vi "Search for Home (SubVI).vi"(9 "Home Mode":T1, 10 "Axis":i32, 11 ".NET Refnum in":refnum<k24>) -> (0 "error out":errorcluster)   [LabVIEW 2019, in "ESP301.lvlib"]
uses:
  ESP301.lvlib
  Newport.ESP301.CommandInterface
  Home Mode.ctl
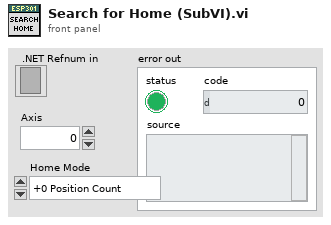
[diagram p1: front panel]
types:
  T1 = typedef "ESP301.lvlib/Home Mode.ctl" = enum16{"+0 Position Count", "Home and Index Singals", "Home Signal", "Positive Limit Signal", "Negative Limit Signal", "Positive Limit Signal and Index Signals", "Negative Limit Signal and Index Signals"}
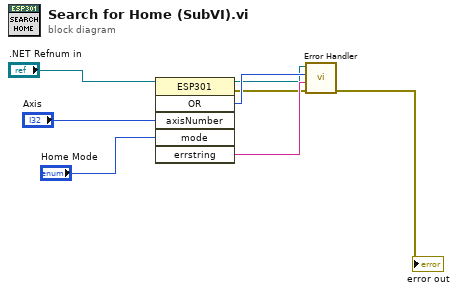
[diagram p0: block diagram]
diagram:
  n1 = invoke class="ESP301" method="OR"(reference=".NET Refnum in", "axisNumber"="Axis", "mode"="Home Mode") -> (reference out=w6:refnum<k24>, error out=w3:errorcluster, "OR"=w7:i32, "errstring"=w8:string)  [unwired: 3 in, 2 out]
  n2 = call "Error Handler.vi"("error in (no error)"=w3, "value"=w8, "OpenInstrument"=w7, ".NET Refnum in"=w6) -> ("error out"=→"error out":errorcluster)  [unwired: 6 in, 1 out]
